vi "历史故障数据读取-V1.0.2.vi"() -> ()   [LabVIEW 2013]
uses:
  SxsenderClassLibrary.dll
  EHCL.dll
panel:
  in  "布尔 3":bool
  out "清故障标志位":i32=2
  out "清历史标志位":i32=2
  out "故障标志位":i32=2
  out "历史标志位":i32=2
  in  "布尔 2":bool
  out "下拉列表":u16(ring) items=["空状态", "读历史", "读故障", "清历史", "清故障"]
  out "Connected":bool
  out "EHCL":refnum<k24>
  in  "读历史数据":bool
  in  "整车CAN测试":bool
  in  "整车CAN测试":bool
  in  "整车CAN测试":bool
  in  "整车CAN测试":bool
  out "x/y":dbl format="%.1f"
  out "引用输出":refnum<k24>
  in  "布尔":bool
  in  "停止":bool
  out "错误输出":errorcluster
  in  "停止":bool
  out "字符串":string
  in  "结果":i32(listbox)=-1
  out "Schedule":u8(slide) scale=0.0..100.0
  in  "波特率":u16(ring)=500 caption="Baudrate" items=["5Kbps"=5, "10Kbps"=10, "20Kbps"=20, "40Kbps"=40, "50Kbps"=50, "80Kbps"=80, "100Kbps"=100, "125Kbps"=125, "200Kbps"=200, "250Kbps"=250, "400Kbps"=400, "500Kbps"=500, "666Kbps"=666, "800Kbps"=800, "1000Kbps"=1000]
  out "Save File Path(Automatic)":path
  in  "CAN端口":u16(ring) caption="CANIndex" items=["0", "1"]
  in  "设备索引号":u16(ring) caption="DevIndex" items=["0", "1", "2", "3", "4", "5", "6", "7", "8", "9", "10", "11", "12", "13", "14", "15", "16"]
  # "历史数据读取上位机"
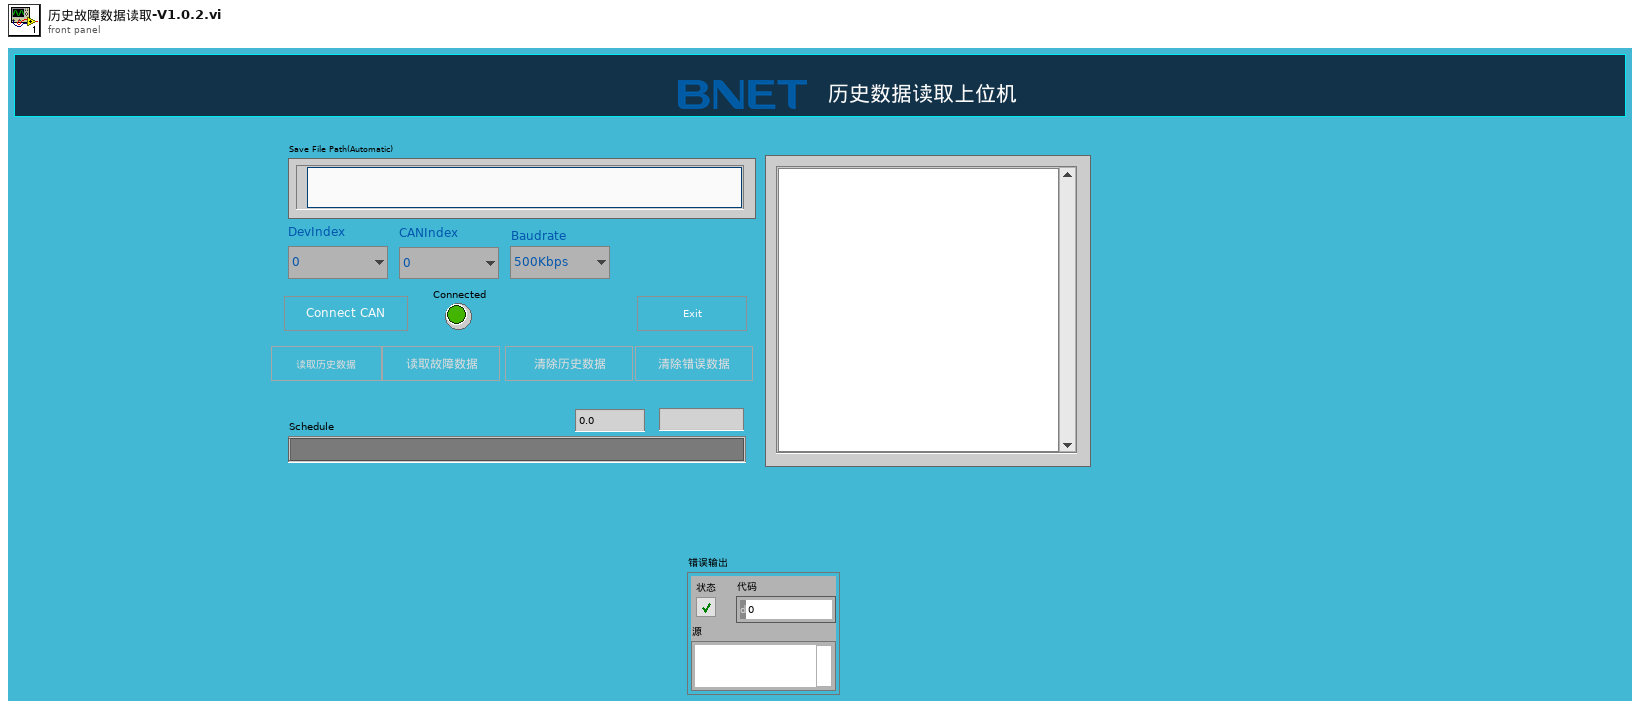
[diagram p1: front panel]
types:
  T1 = enum32{"Invalid", "Standard", "Closed", "Hidden", "Minimized", "Maximized"}
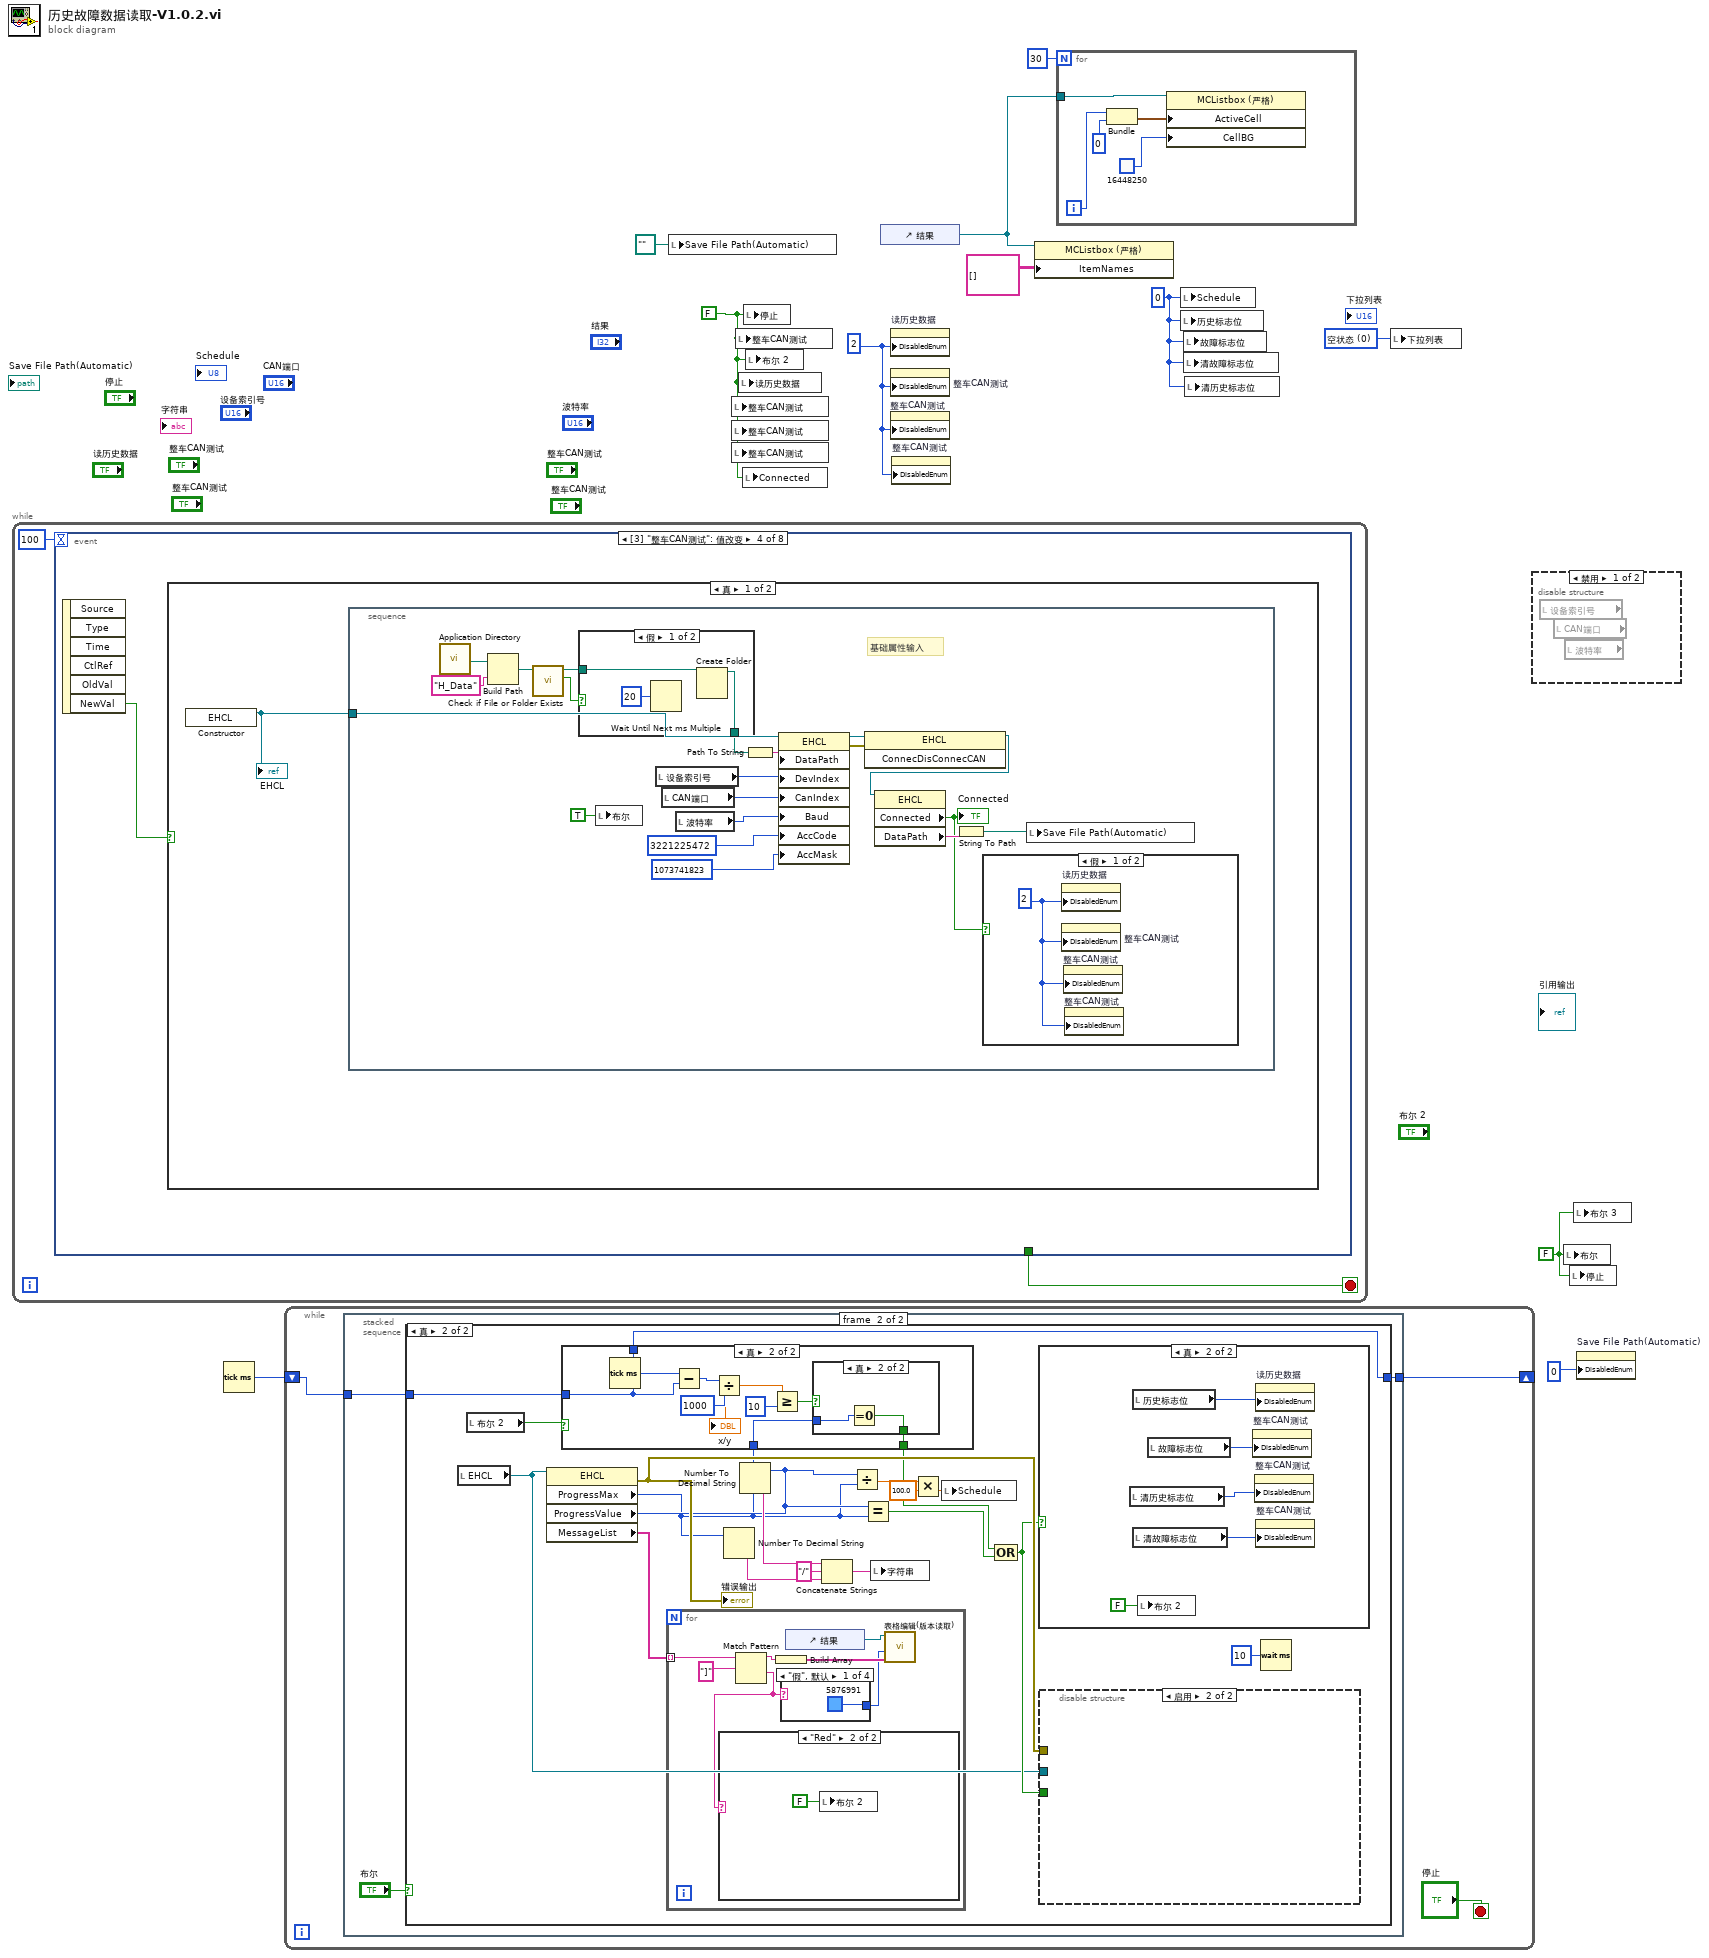
[diagram p0: block diagram]
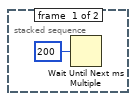
[diagram p3: hidden frame]
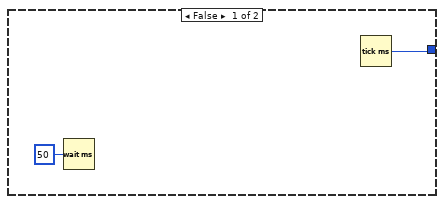
[diagram p4: hidden frame]
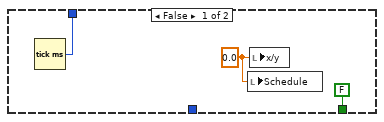
[diagram p5: hidden frame]
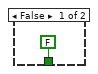
[diagram p6: hidden frame]
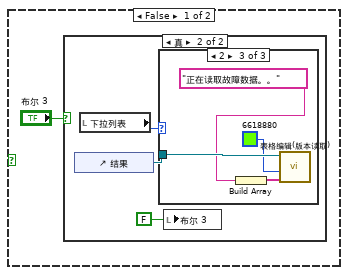
[diagram p7: hidden frame]
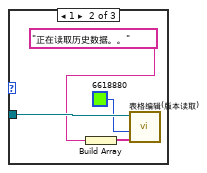
[diagram p10: hidden frame]
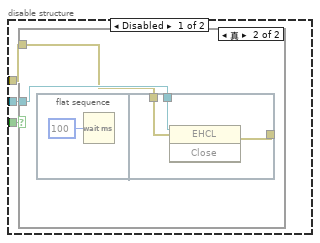
[diagram p11: hidden frame]
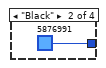
[diagram p14: hidden frame]
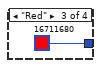
[diagram p15: hidden frame]
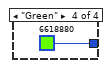
[diagram p16: hidden frame]
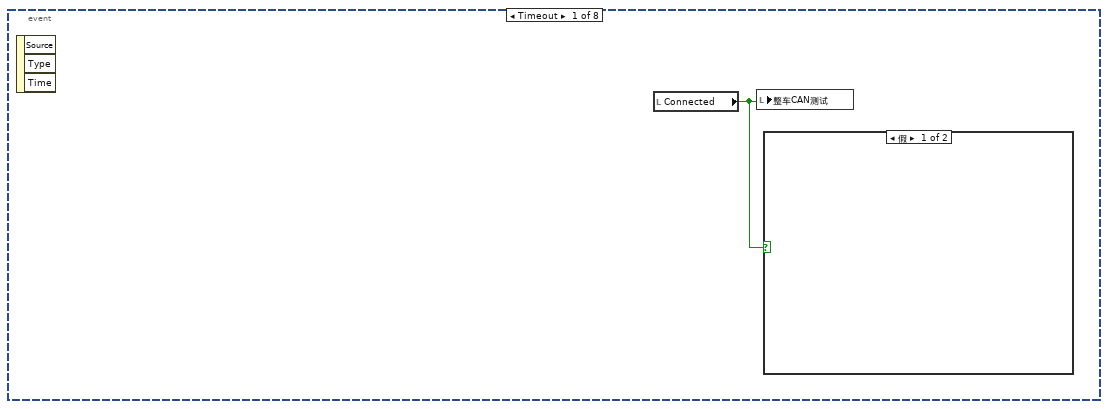
[diagram p17: hidden frame]
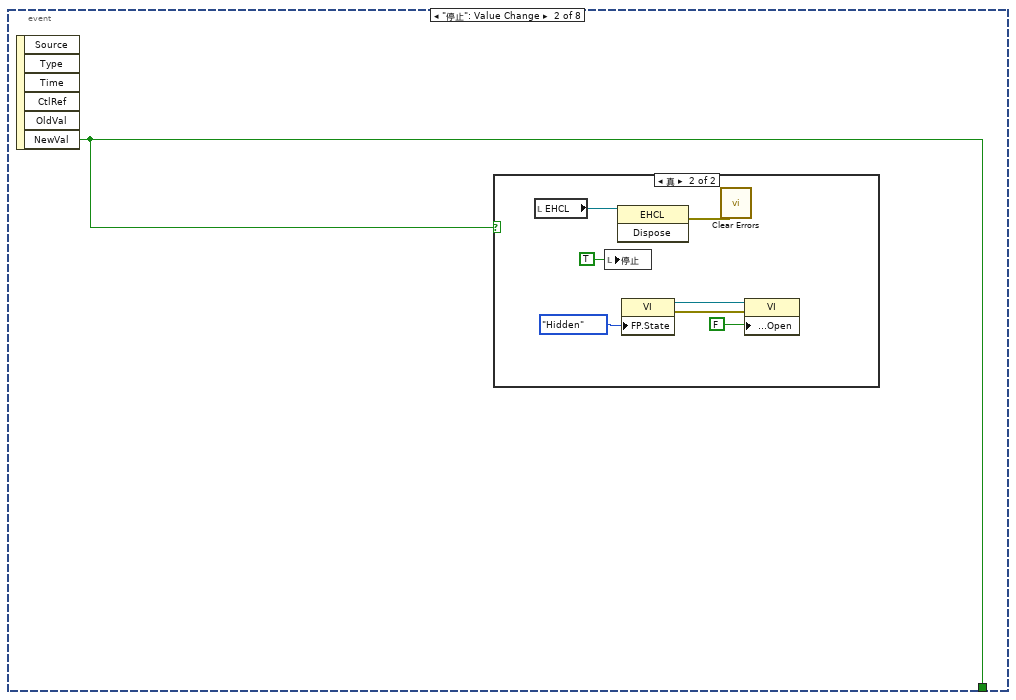
[diagram p19: hidden frame]
diagram:
  w2 = u16 0 items=["空状态", "读历史", "读故障", "清历史", "清故障"] ("下拉列表")
  w1 = FALSE ("布尔")
  w4 = u8 0 ("刷写进度")
  w3 = FALSE ("开始刷写")
  w5 = 2
  n1 = while {
    stop <- w13 stop-if-true
    n2 = event shown="[3] \"整车CAN测试\": 值改变" {
      selector: _ -> [_ _ _ _ _ _ _ _]
      dyn-events: _ -> [_ _ _ _ _ _ _ _]
      timeout: 100 -> [_ _ _ _ _ _ _ _]
      tunnel: [_ w15 w23 _ _ _ _ _] -> w13
      event Timeout {
        n3 = event-data() -> ()  [unwired: 1 in, 3 out]
        n4 = local read "Connected"() -> (w14:bool)
        n5 = local write "整车CAN测试"(w14) -> ()
        n6 = case shown="假" w14 {
          frame False {
          }
          frame True {
          }
        }
      }
      event "停止": Value Change {
        n7 = event-data() -> ("NewVal"=w15:bool)  [unwired: 1 in, 5 out]
        n8 = case shown="真" w15 {
          frame False {
          }
          frame True {
            n9 = local read "EHCL"() -> (w22:refnum<k24>)
            n10 = local write "停止"(TRUE ("停止")) -> ()
            n11 = invoke on="调用节点" class="EHCL" method="Dispose"(reference=w22) -> (error out=w16:errorcluster)  [unwired: 2 in, 2 out]
            n12 = property class="VI"("FP.State"=T1."Hidden" ("前面板窗口:状态")) -> (reference out=w18:refnum<vi>, error out=w17:errorcluster)  [unwired: 2 in]
            n13 = call <vilib>:"Clear Errors.vi"("error in (no error)"=w16) -> ()  [unwired: 6 in, 1 out]
            n14 = property class="VI"(reference=w18, error in=w17, "Front Panel.Open"=FALSE ("前面板窗口:打开")) -> ()  [unwired: 2 out]
          }
        }
      }
      event Panel Close? {
        w23 = TRUE
        n15 = event-data() -> ()  [unwired: 1 in, 4 out]
        n16 = case shown="真" w23 {
          frame False {
          }
          frame True {
            n17 = local read "EHCL"() -> (w30:refnum<k24>)
            n18 = local write "停止"(TRUE ("停止")) -> ()
            n19 = property class="VI"("FP.State"=T1."Hidden" ("前面板窗口:状态")) -> (reference out=w26:refnum<vi>, error out=w25:errorcluster)  [unwired: 2 in]
            n20 = invoke on="调用节点" class="EHCL" method="Dispose"(reference=w30) -> (error out=w24:errorcluster)  [unwired: 2 in, 2 out]
            n21 = call <vilib>:"Clear Errors.vi"("error in (no error)"=w24) -> ()  [unwired: 6 in, 1 out]
            n22 = property class="VI"(reference=w26, error in=w25, "Front Panel.Open"=FALSE ("前面板窗口:打开")) -> ()  [unwired: 2 out]
          }
        }
        n23 = event-data("Discard?"=w23) -> ()  [unwired: 1 in, 1 out]
      }
      event "整车CAN测试": Value Change {
        n24 = event-data() -> ("NewVal"=w31:bool)  [unwired: 1 in, 5 out]
        n25 = case shown="真" w31 {
          frame True {
            n26 = constructor class="EHCL"() -> (reference out=w32:refnum<k24>)  [unwired: 3 in, 2 out]
            "EHCL" <- w32
            n27 = stacked-sequence {
              tunnel: w32 -> [w52]
              frame #0 {
                # "基础属性输入"
                n28 = call <vilib>:"Application Directory.vi"() -> ("Application Directory"=w41:path)
                n29 = Build Path(base path=w41, name or relative path="H_Data" ("名称或相对路径")) -> (appended path=w39:path)
                n30 = call <vilib>:"Check if File or Folder Exists.vi"("path"=w39) -> ("file or folder exists?"=w38:bool, "dup path"=w37:path)  [unwired: 8 in, 1 out]
                n31 = case shown="假" w38 {
                  tunnel: [w55 w56] -> w42
                  tunnel: w37 -> [w54 w56]
                  frame False {
                    n32 = Wait Until Next ms Multiple(millisecond multiple=u32 20 ("毫秒倍数")) -> ()  [unwired: 1 out]
                    n33 = Create Folder(path (use dialog)=w54) -> (created path=w55:path)  [unwired: 2 in, 2 out]
                  }
                  frame True {
                  }
                }
                n34 = local write "布尔"(TRUE ("布尔")) -> ()
                n35 = local read "设备索引号"() -> (w49:u16)
                n36 = local read "CAN端口"() -> (w48:u16)
                n37 = local read "波特率"() -> (w50:u16)
                n38 = Path To String(path=w42) -> (string=w51:string)
                n39 = property on="属性节点" class="EHCL"(reference=w52, "DataPath"=w51, "DevIndex"=w49, "CanIndex"=w48, "Baud"=w50, "AccCode"=u32 3221225472 ("Accept Code"), "AccMask"=u32 1073741823 ("Accept Code")) -> (reference out=w47:refnum<k24>, error out=w46:errorcluster)  [unwired: 1 in]
                n40 = invoke on="调用节点" class="EHCL" method="ConnecDisConnecCAN"(reference=w47, error in=w46) -> (reference out=w36:refnum<k24>)  [unwired: 1 in, 2 out]
                n41 = property on="属性节点" class="EHCL"(reference=w36) -> ("Connected"=w43:bool, "DataPath"=w45:string)  [unwired: 1 in, 2 out]
                "Connected" <- w43
                n42 = String To Path(string=w45) -> (path=w44:path)
                n43 = case shown="假" w43 {
                  frame False {
                    w57 = 2
                    n44 = property on="读历史数据" class="Bool (严格)"("DisabledEnum"=w57) -> ()  [unwired: 2 in, 2 out]
                    n45 = property on="整车CAN测试" class="Bool (严格)"("DisabledEnum"=w57) -> ()  [unwired: 2 in, 2 out]
                    n46 = property on="整车CAN测试" class="Bool (严格)"("DisabledEnum"=w57) -> ()  [unwired: 2 in, 2 out]
                    n47 = property on="整车CAN测试" class="Bool (严格)"("DisabledEnum"=w57) -> ()  [unwired: 2 in, 2 out]
                  }
                  frame True {
                    w58 = 0
                    n48 = property on="读历史数据" class="Bool (严格)"("DisabledEnum"=w58) -> ()  [unwired: 2 in, 2 out]
                    n49 = property on="整车CAN测试" class="Bool (严格)"("DisabledEnum"=w58) -> ()  [unwired: 2 in, 2 out]
                    n50 = property on="整车CAN测试" class="Bool (严格)"("DisabledEnum"=w58) -> ()  [unwired: 2 in, 2 out]
                    n51 = property on="整车CAN测试" class="Bool (严格)"("DisabledEnum"=w58) -> ()  [unwired: 2 in, 2 out]
                  }
                }
                n52 = local write "Save File Path(Automatic)"(w44) -> ()
              }
            }
          }
          frame False {
            n53 = stacked-sequence {
              frame #0 {
                # "基础属性输入"
                n54 = local read "EHCL"() -> (w60:refnum<k24>)
                n55 = invoke on="调用节点" class="EHCL" method="ConnecDisConnecCAN"(reference=w60) -> (reference out=w61:refnum<k24>)  [unwired: 2 in, 2 out]
                n56 = property on="属性节点" class="EHCL"(reference=w61) -> ("Connected"=w59:bool)  [unwired: 1 in, 2 out]
                n57 = local write "Connected"(w59) -> ()
                n58 = case shown="假" w59 {
                  frame False {
                    w62 = 2
                    n59 = property on="读历史数据" class="Bool (严格)"("DisabledEnum"=w62) -> ()  [unwired: 2 in, 2 out]
                    n60 = property on="整车CAN测试" class="Bool (严格)"("DisabledEnum"=w62) -> ()  [unwired: 2 in, 2 out]
                    n61 = property on="整车CAN测试" class="Bool (严格)"("DisabledEnum"=w62) -> ()  [unwired: 2 in, 2 out]
                    n62 = property on="整车CAN测试" class="Bool (严格)"("DisabledEnum"=w62) -> ()  [unwired: 2 in, 2 out]
                  }
                  frame True {
                  }
                }
              }
            }
          }
        }
      }
      event "读历史数据": Value Change {
        n63 = event-data() -> ("NewVal"=w63:bool)  [unwired: 1 in, 5 out]
        n64 = case shown="真" w63 {
          frame False {
          }
          frame True {
            w65 = 2
            n65 = stacked-sequence {
              tunnel: [w69] -> w66
              frame #0 {
                w68 = u16 1 items=["空状态", "读历史", "读故障", "清历史", "清故障"] ("下拉列表")
                n66 = local write "下拉列表"(w68) -> ()
                n67 = local read "EHCL"() -> (w69:refnum<k24>)
                "历史标志位" <- 2 ("历史标志位")
              }
            }
            n68 = invoke on="调用节点" class="EHCL" method="ReadHistoryInfor"(reference=w66) -> (reference out=w64:refnum<k24>)  [unwired: 2 in, 2 out]
            n69 = property on="读历史数据" class="Bool (严格)"("DisabledEnum"=w65) -> ()  [unwired: 2 in, 2 out]
            n70 = property on="整车CAN测试" class="Bool (严格)"("DisabledEnum"=w65) -> ()  [unwired: 2 in, 2 out]
            n71 = property on="整车CAN测试" class="Bool (严格)"("DisabledEnum"=w65) -> ()  [unwired: 2 in, 2 out]
            n72 = property on="整车CAN测试" class="Bool (严格)"("DisabledEnum"=w65) -> ()  [unwired: 2 in, 2 out]
            n73 = stacked-sequence {
              tunnel: w64 -> [_ _]
              frame #0 {
                n74 = Wait Until Next ms Multiple(millisecond multiple=u32 50 ("毫秒倍数")) -> ()  [unwired: 1 out]
              }
              frame #1 {
                w71 = TRUE ("布尔 2")
                n75 = local write "布尔 2"(w71) -> ()
                n76 = local write "布尔 3"(w71) -> ()
              }
            }
          }
        }
      }
      event "整车CAN测试": Value Change {
        n77 = event-data() -> ("NewVal"=w72:bool)  [unwired: 1 in, 5 out]
        n78 = case shown="真" w72 {
          frame False {
          }
          frame True {
            w74 = 2
            n79 = stacked-sequence {
              tunnel: [w78] -> w75
              frame #0 {
                w76 = u16 2 items=["空状态", "读历史", "读故障", "清历史", "清故障"] ("下拉列表")
                n80 = local write "下拉列表"(w76) -> ()
                n81 = local read "EHCL"() -> (w78:refnum<k24>)
                "故障标志位" <- 2 ("历史标志位")
              }
            }
            n82 = invoke on="调用节点" class="EHCL" method="ReadErrorInfor"(reference=w75) -> (reference out=w73:refnum<k24>)  [unwired: 2 in, 2 out]
            n83 = property on="读历史数据" class="Bool (严格)"("DisabledEnum"=w74) -> ()  [unwired: 2 in, 2 out]
            n84 = property on="整车CAN测试" class="Bool (严格)"("DisabledEnum"=w74) -> ()  [unwired: 2 in, 2 out]
            n85 = property on="整车CAN测试" class="Bool (严格)"("DisabledEnum"=w74) -> ()  [unwired: 2 in, 2 out]
            n86 = property on="整车CAN测试" class="Bool (严格)"("DisabledEnum"=w74) -> ()  [unwired: 2 in, 2 out]
            n87 = stacked-sequence {
              tunnel: w73 -> [_ _]
              frame #0 {
                n88 = Wait Until Next ms Multiple(millisecond multiple=u32 50 ("毫秒倍数")) -> ()  [unwired: 1 out]
              }
              frame #1 {
                w80 = TRUE ("布尔 2")
                n89 = local write "布尔 2"(w80) -> ()
                n90 = local write "布尔 3"(w80) -> ()
              }
            }
          }
        }
      }
      event "整车CAN测试": Value Change {
        n91 = event-data() -> ("NewVal"=w81:bool)  [unwired: 1 in, 5 out]
        n92 = case shown="真" w81 {
          frame False {
          }
          frame True {
            n93 = local read "EHCL"() -> (w82:refnum<k24>)
            n94 = invoke on="调用节点" class="EHCL" method="ClearHistoryInfor"(reference=w82) -> ()  [unwired: 2 in, 3 out]
            n95 = property on="整车CAN测试" class="Bool (严格)"("DisabledEnum"=2) -> ()  [unwired: 2 in, 2 out]
            "清历史标志位" <- 2 ("历史标志位")
          }
        }
      }
      event "整车CAN测试": Value Change {
        n96 = event-data() -> ("NewVal"=w85:bool)  [unwired: 1 in, 5 out]
        n97 = case shown="真" w85 {
          frame False {
          }
          frame True {
            n98 = local read "EHCL"() -> (w86:refnum<k24>)
            n99 = invoke on="调用节点" class="EHCL" method="ClearErrorInfor"(reference=w86) -> ()  [unwired: 2 in, 3 out]
            n100 = property on="整车CAN测试" class="Bool (严格)"("DisabledEnum"=2) -> ()  [unwired: 2 in, 2 out]
            "清故障标志位" <- 2 ("历史标志位")
          }
        }
      }
    }
  }
  n101 = Tick Count (ms)() -> (millisecond timer value=w7:u32)
  n102 = while {
    shift-right: [w90] -> _
    shift-left: w7 -> [w89]
    stop <- "停止" stop-if-true
    n103 = stacked-sequence {
      tunnel: [_ w94] -> w90
      tunnel: w89 -> [_ w93]
      frame #0 {
        n104 = Wait Until Next ms Multiple(millisecond multiple=u32 200 ("毫秒倍数")) -> ()  [unwired: 1 out]
      }
      frame #1 {
        n105 = case shown="真" "布尔" {
          tunnel: [w96 w100] -> w94
          tunnel: w93 -> [_ w102]
          frame False {
            n106 = Wait (ms)(milliseconds to wait=u32 50 ("等待时间（毫秒）")) -> ()  [unwired: 1 out]
            n107 = Tick Count (ms)() -> (millisecond timer value=w96:u32)
          }
          frame True {
            n108 = local read "EHCL"() -> (w99:refnum<k24>)
            n109 = local read "布尔 2"() -> (w98:bool)
            n110 = property on="属性节点" class="EHCL"(reference=w99) -> (error out=w107:errorcluster, "ProgressMax"=w104:u32, "ProgressValue"=w106:u32, "MessageList"=w108:string[])  [unwired: 1 in, 1 out]
            "错误输出" <- w107
            n111 = case shown="真" w98 {
              tunnel: w104 -> [_ w122]
              tunnel: [FALSE w121] -> w103
              tunnel: w102 -> [_ w120]
              tunnel: [w118 w120] -> w100
              frame False {
                w117 = 0.0 ("x/y")
                n112 = Tick Count (ms)() -> (millisecond timer value=w118:u32)
                n113 = local write "Schedule"(w117) -> ()
                n114 = local write "x/y"(w117) -> ()
              }
              frame True {
                n115 = Tick Count (ms)() -> (millisecond timer value=w128:u32)
                n116 = Subtract(x=w128, y=w120) -> (x-y=w127:u32)
                n117 = Divide(x=w127, y=u32 1000) -> (x/y=w125:dbl)
                "x/y" <- w125
                n118 = Greater Or Equal?(x=w125, y=u32 10) -> (x >= y?=w123:bool)
                n119 = case shown="真" w123 {
                  tunnel: w122 -> [_ w131]
                  tunnel: [FALSE w130] -> w121
                  frame False {
                  }
                  frame True {
                    n120 = Equal To 0?(x=w131) -> (x = 0?=w130:bool)
                  }
                }
              }
            }
            n121 = for {
              tunnel: w108 -> [w160] mode=indexing
              n122 = Match Pattern(string=w160, regular expression="]") -> (before substring=w163:string, after substring=w159:string)  [unwired: 1 in, 2 out]
              n123 = case shown="\"Red\"" w159 {
                frame "假", Default {
                }
                frame "Red" {
                  n124 = local write "布尔 2"(FALSE ("布尔 2")) -> ()
                }
              }
              n125 = Build Array(w163) -> (w162:string[])
              n126 = case shown="\"假\", 默认" w159 {
                tunnel: [u32 5876991 u32 5876991 u32 16711680 u32 6618880] -> w161
                frame "假", Default {
                }
                frame "Black" {
                }
                frame "Red" {
                }
                frame "Green" {
                }
              }
              n127 = control-ref of="结果"() -> (w158:refnum<vi>)
              n128 = call "表格编辑(版本读取).vi"("新元素/子数组"=w162, "活动单元格:单元格背景色"=w161, "MCListbox引用句柄"=w158) -> ()  [unwired: 9 in]
            }
            n129 = Number To Decimal String(number=w104) -> (decimal integer string=w112:string)  [unwired: 1 in]
            n130 = Number To Decimal String(number=w106) -> (decimal integer string=w111:string)  [unwired: 1 in]
            n131 = Concatenate Strings(w111, "/" ("字符串"), w112) -> (w109:string)
            n132 = Divide(x=w106, y=w104) -> (x/y=w115:dbl)
            n133 = Equal?(x=w106, y=w104) -> (x = y?=w116:bool)
            n134 = local write "字符串"(w109) -> ()
            n135 = Multiply(x=w115, y=100.0) -> (x*y=w113:dbl)
            n136 = local write "Schedule"(w113) -> ()
            n137 = Compound Arithmetic op=OR(w103, w116) -> (w101:bool)
            n138 = case shown="真" w101 {
              frame False {
                n139 = case shown="真" "布尔 3" {
                  frame False {
                  }
                  frame True {
                    n140 = control-ref of="结果"() -> (w134:refnum<vi>)
                    n141 = local read "下拉列表"() -> (w135:u16)
                    n142 = case shown="2" w135 {
                      tunnel: w134 -> [_ w139 w143]
                      frame 0, Default {
                      }
                      frame 1 {
                        n143 = Build Array("正在读取历史数据。。") -> (w138:string[])
                        n144 = call "表格编辑(版本读取).vi"("新元素/子数组"=w138, "活动单元格:单元格背景色"=u32 6618880, "MCListbox引用句柄"=w139) -> ()  [unwired: 9 in]
                      }
                      frame 2 {
                        n145 = Build Array("正在读取故障数据。。") -> (w142:string[])
                        n146 = call "表格编辑(版本读取).vi"("新元素/子数组"=w142, "活动单元格:单元格背景色"=u32 6618880, "MCListbox引用句柄"=w143) -> ()  [unwired: 9 in]
                      }
                    }
                    n147 = local write "布尔 3"(FALSE ("布尔 3")) -> ()
                  }
                }
              }
              frame True {
                n148 = local read "清历史标志位"() -> (w144:i32)
                n149 = local read "历史标志位"() -> (w147:i32)
                n150 = local read "清故障标志位"() -> (w145:i32)
                n151 = local write "布尔 2"(FALSE ("布尔 2")) -> ()
                n152 = local read "故障标志位"() -> (w146:i32)
                n153 = property on="整车CAN测试" class="Bool (严格)"("DisabledEnum"=w146) -> ()  [unwired: 2 in, 2 out]
                n154 = property on="整车CAN测试" class="Bool (严格)"("DisabledEnum"=w144) -> ()  [unwired: 2 in, 2 out]
                n155 = property on="读历史数据" class="Bool (严格)"("DisabledEnum"=w147) -> ()  [unwired: 2 in, 2 out]
                n156 = property on="整车CAN测试" class="Bool (严格)"("DisabledEnum"=w145) -> ()  [unwired: 2 in, 2 out]
              }
            }
            n157 = disable-structure shown="启用" {
              disable-tunnel: w101 -> [w151 _]
              disable-tunnel: w99 -> [w150 _]
              disable-tunnel: w107 -> [w149 _]
              frame Disabled {
                n158 = case shown="真" w151 {
                  tunnel: w150 -> [_ w153]
                  tunnel: w149 -> [_ w152]
                  frame False {
                  }
                  frame True {
                    n159 = flat-sequence {
                      tunnel: w152 -> [w156]
                      tunnel: [w157] -> _
                      tunnel: w153 -> [w155]
                      frame #0 {
                        n160 = Wait (ms)(milliseconds to wait=u32 100 ("等待时间（毫秒）")) -> ()  [unwired: 1 out]
                      }
                      frame #1 {
                        n161 = invoke class="EHCL" method="Close"(reference=w155, error in=w156) -> (error out=w157:errorcluster)  [unwired: 1 in, 2 out]
                      }
                    }
                  }
                }
              }
              frame Enabled {
              }
            }
            n162 = Wait (ms)(milliseconds to wait=u32 10 ("等待时间（毫秒）")) -> ()  [unwired: 1 out]
          }
        }
      }
    }
  }
  n163 = local write "Save File Path(Automatic)"(path "" ("SX文件路径")) -> ()
  n164 = local write "整车CAN测试"(w3) -> ()
  n165 = local write "整车CAN测试"(w3) -> ()
  n166 = local write "整车CAN测试"(w3) -> ()
  n167 = local write "整车CAN测试"(w3) -> ()
  n168 = local write "读历史数据"(w3) -> ()
  n169 = local write "Connected"(w3) -> ()
  n170 = local write "停止"(w3) -> ()
  n171 = local write "布尔 2"(w3) -> ()
  n172 = control-ref of="结果"() -> (w9:refnum<vi>)
  n173 = property on="读历史数据" class="Bool (严格)"("DisabledEnum"=w5) -> ()  [unwired: 2 in, 2 out]
  n174 = property on="整车CAN测试" class="Bool (严格)"("DisabledEnum"=w5) -> ()  [unwired: 2 in, 2 out]
  n175 = property on="整车CAN测试" class="Bool (严格)"("DisabledEnum"=w5) -> ()  [unwired: 2 in, 2 out]
  n176 = property on="整车CAN测试" class="Bool (严格)"("DisabledEnum"=w5) -> ()  [unwired: 2 in, 2 out]
  n177 = property class="MCListbox (严格)"(reference=w9, "ItemNames"=string[][] [] ("项名")) -> ()  [unwired: 1 in, 2 out]
  n178 = for {
    N: 30 -> [_]
    tunnel: w9 -> [w174]
    i -> [w171]
    n179 = Bundle(w171, 0) -> (w173:cluster{i32, i32})  [unwired: 1 out]
    n180 = property class="MCListbox (严格)"(reference=w174, "ActiveCell"=w173, "CellBG"=u32 16448250) -> ()  [unwired: 1 in, 2 out]
  }
  n181 = local write "Schedule"(w4) -> ()
  n182 = local write "历史标志位"(w4) -> ()
  n183 = local write "故障标志位"(w4) -> ()
  n184 = local write "清故障标志位"(w4) -> ()
  n185 = local write "清历史标志位"(w4) -> ()
  n186 = local write "下拉列表"(w2) -> ()
  n187 = disable-structure shown="禁用" {
    frame Disabled {
      n188 = local read "设备索引号"() -> ()  [unwired: 1 out]
      n189 = local read "CAN端口"() -> ()  [unwired: 1 out]
      n190 = local read "波特率"() -> ()  [unwired: 1 out]
    }
    frame Enabled {
    }
  }
  n191 = local write "布尔"(w1) -> ()
  n192 = local write "停止"(w1) -> ()
  n193 = local write "布尔 3"(w1) -> ()
  n194 = property on="Save File Path(Automatic)" class="Path"("DisabledEnum"=0) -> ()  [unwired: 2 in, 2 out]
